vi "Config Curve Point.vi"(0 "VISA resource name":refnum<visa-resource-name>, 5 "Curve (1)":dbl=1.0 min=1.0 max=20.0 step=1.0, 7 "Index (1)":dbl=1.0 min=1.0 max=200.0 step=1.0, 9 "Temperature Value (0.0000)":dbl min=-9999.0 max=9999.0 step=1e-05 format="%.4f", 11 "error in (no error)":errorcluster, 12 "Units Value (0.00000)":dbl min=-9999.0 max=9999.0 step=1e-05 format="%.5f") -> (4 "VISA resource name out":refnum<visa-resource-name>, 15 "error out":errorcluster)   [LabVIEW 2012, in "Lake Shore Cryotronics 370.lvlib"]
doc: "This VI Configures a user curve point."
uses:
  <instrlib>/Lake Shore Cryotronics 370/Lake Shore Cryotronics 370.lvlib
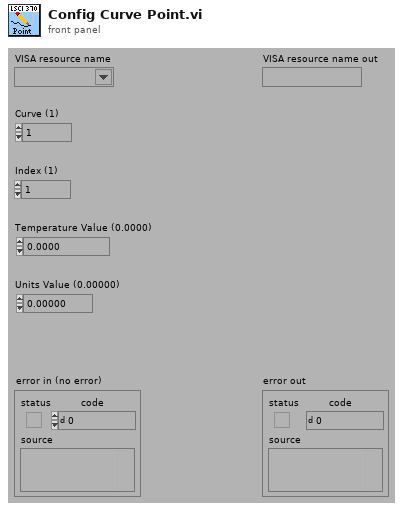
[diagram p1: front panel]
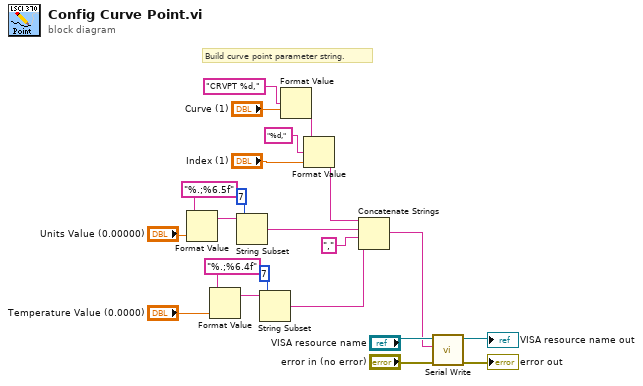
[diagram p0: block diagram]
diagram:
  # "Build curve point parameter string."
  n1 = Format Value(format string="%.;%6.5f", value (0)="Units Value (0.00000)") -> (output string=w16:string)  [unwired: 1 in]
  n2 = Format Value(format string="%.;%6.4f", value (0)="Temperature Value (0.0000)") -> (output string=w9:string)  [unwired: 1 in]
  n3 = String Subset(string=w16, length (rest)=7) -> (substring=w12:string)  [unwired: 1 in]
  n4 = String Subset(string=w9, length (rest)=7) -> (substring=w6:string)  [unwired: 1 in]
  n5 = Format Value(format string="CRVPT %d,", value (0)="Curve (1)") -> (output string=w19:string)  [unwired: 1 in]
  n6 = Format Value(string ("")=w19, format string="%d,", value (0)="Index (1)") -> (output string=w13:string)
  n7 = Concatenate Strings(w13, w12, ",", w6) -> (w1:string)
  n8 = call <instrlib>:"Serial Write.vi"("error in (no error)"="error in (no error)", "Write Buffer (\"\")"=w1, "VISA resource name"="VISA resource name") -> ("error out"=→"error out":errorcluster, "VISA resource name out"=→"VISA resource name out":refnum<visa-resource-name>)  [unwired: 6 in, 1 out]
